vi "Create Evaluation String.vi"(8 "error in (no error)":errorcluster, 10 "Evaluation String":string, 11 "Boolean in":refnum<class "Boolean.lvclass">) -> (0 "error out":errorcluster, 3 "Boolean out":refnum<class "Boolean.lvclass">)   [LabVIEW 2018, in "Boolean.lvclass"]
uses:
  Boolean.lvclass
  C:/Users/UKHornP/Documents/Work/Projects/Assert API/Plugins/Utility/Test Classes/Test.lvclass
  03011840-08fb-4e8a-87dd-40cd17e5a716.vi
  <vilib>/JDP Science/JSONtext/JSON text to Variant.vi
  Test.lvclass
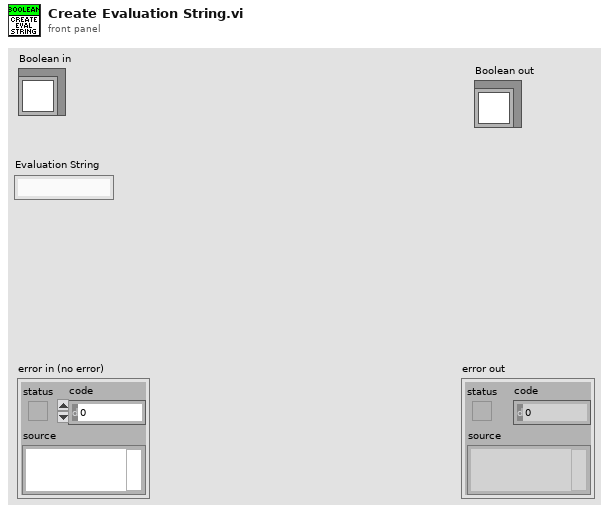
[diagram p1: front panel]
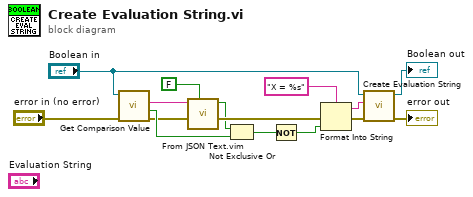
[diagram p0: block diagram]
diagram:
  n1 = call "Get Comparison Value.vi"("error in (no error)"="error in (no error)", "Test in"="Boolean in") -> ("error out"=w1:errorcluster, "Invert Result"=w2:bool, "Data String"=w3:string)  [unwired: 7 in]
  n2 = call "From JSON Text.vim"("Data Type and Default Value"=FALSE, "error in (no error)"=w1, "JSON"=w3) -> ("error out"=w13:errorcluster, "Data out"=w8:bool)  [unwired: 7 in]
  n3 = Not Exclusive Or(1:w2, 2:w8) -> (0:w10:bool)
  n4 = Not(x=w10) -> (.not. x?=w9:bool)
  n5 = Format Into String(format string="X = %s" ("Evaluation String"), error in=w13, w9) -> (resulting string=w6:string, error out=w11:errorcluster)  [unwired: 1 in]
  n6 = call-parent "Create Evaluation String.vi"("error in (no error)"=w11, "Evaluation String"=w6, "Test in"="Boolean in") -> ("error out"=→"error out":errorcluster, "Test out"=→"Boolean out":refnum<class "Boolean.lvclass">)  [unwired: 7 in]
